vi "create board.vi"() -> (0 "2048 2":T1[][](array[typedef]), 3 "board":dbl[][](array[numeric]))   [LabVIEW 2015]
uses:
  colorbox cluster.ctl
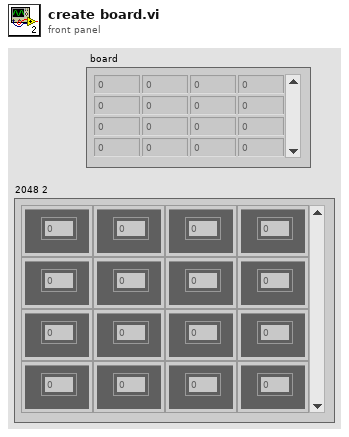
[diagram p1: front panel]
types:
  T1 = typedef "colorbox cluster.ctl" = cluster{"Color Box":u32, "Numeric":dbl}
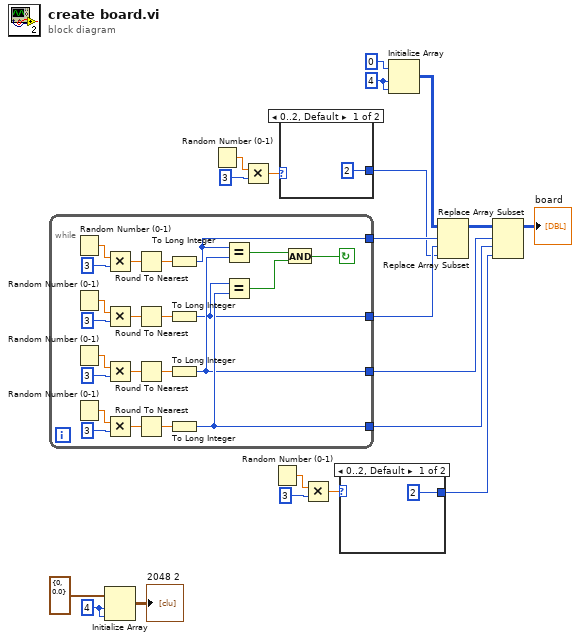
[diagram p0: block diagram]
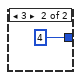
[diagram p2: hidden frame]
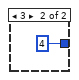
[diagram p3: hidden frame]
diagram:
  w2 = 4
  w20 = 4
  n1 = while {
    tunnel: [w24] -> w11
    tunnel: [w22] -> w7
    tunnel: [w21] -> w10
    tunnel: [w23] -> w6
    stop <- w25 continue-if-true
    n2 = Random Number (0-1)() -> (number: 0 to 1=w38:dbl)
    n3 = Random Number (0-1)() -> (number: 0 to 1=w33:dbl)
    n4 = Random Number (0-1)() -> (number: 0 to 1=w41:dbl)
    n5 = Random Number (0-1)() -> (number: 0 to 1=w30:dbl)
    n6 = Multiply(x=w38, y=3) -> (x*y=w36:dbl)
    n7 = Multiply(x=w33, y=3) -> (x*y=w35:dbl)
    n8 = Multiply(x=w41, y=3) -> (x*y=w43:dbl)
    n9 = Multiply(x=w30, y=3) -> (x*y=w28:dbl)
    n10 = Round To Nearest(number=w36) -> (nearest integer value=w39:dbl)
    n11 = Round To Nearest(number=w35) -> (nearest integer value=w32:dbl)
    n12 = Round To Nearest(number=w43) -> (nearest integer value=w40:dbl)
    n13 = Round To Nearest(number=w28) -> (nearest integer value=w31:dbl)
    n14 = To Long Integer(number=w39) -> (32bit integer=w24:i32)
    n15 = To Long Integer(number=w32) -> (32bit integer=w21:i32)
    n16 = To Long Integer(number=w40) -> (32bit integer=w22:i32)
    n17 = To Long Integer(number=w31) -> (32bit integer=w23:i32)
    n18 = Equal?(x=w24, y=w22) -> (x = y?=w27:bool)
    n19 = Equal?(x=w21, y=w23) -> (x = y?=w26:bool)
    n20 = And(x=w27, y=w26) -> (x .and. y?=w25:bool)
  }
  n21 = Initialize Array(T1 {"Color Box"=0, "Numeric"=0.0} ("Cluster"), w2, w2) -> (→"2048 2":T1[][])
  n22 = Random Number (0-1)() -> (number: 0 to 1=w18:dbl)
  n23 = Multiply(x=w18, y=3) -> (x*y=w16:dbl)
  n24 = Random Number (0-1)() -> (number: 0 to 1=w13:dbl)
  n25 = case shown="0..2, Default" w16 {
    tunnel: [2 4] -> w9
    frame 0..2, Default {
    }
    frame 3 {
    }
  }
  n26 = Multiply(x=w13, y=3) -> (x*y=w15:dbl)
  n27 = case shown="0..2, Default" w15 {
    tunnel: [2 4] -> w5
    frame 0..2, Default {
    }
    frame 3 {
    }
  }
  n28 = Initialize Array(0, w20, w20) -> (w12:i32[][])
  n29 = Replace Array Subset(array=w12, new element=w9, index (row)=w11, index (col)=w10) -> (w8:i32[][])
  n30 = Replace Array Subset(array=w8, new element=w5, index (row)=w7, index (col)=w6) -> (→"board":i32[][])
